vi "Strip Test Name from Tree GUID.vi"(1 "TestTag GUID":string) -> (0 "Test GUID":string)   [LabVIEW 2011, in "GraphicalTestRunner.lvlib"]
uses:
  GraphicalTestRunner.lvlib
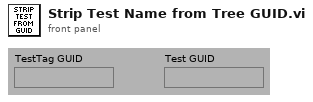
[diagram p1: front panel]
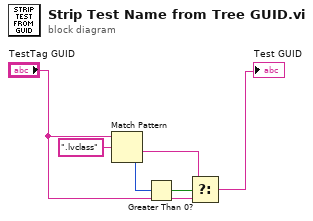
[diagram p0: block diagram]
diagram:
  n1 = Match Pattern(string="TestTag GUID", regular expression=".lvclass") -> (after substring=w5:string, offset past match=w2:i32)  [unwired: 1 in, 2 out]
  n2 = Greater Than 0?(x=w2) -> (x > 0?=w3:bool)
  n3 = Select(t=w5, s=w3, f="TestTag GUID") -> (s? t:f=→"Test GUID":string)
